vi "YAFFooter_TemplateMethod.vi"(8 "ErrorIn":errorcluster, 10 "CmdData":variant, 11 "YAFFooter:YAFFooter in":refnum<class>) -> (0 "ErrorOut":errorcluster, 2 "ReplyData":variant, 3 "YAFFooter:YAFFooter out":refnum<class>, 4 "Exit":bool)   [LabVIEW 2021, in "YAFFooter.lvlib" / "YAFFooter.lvclass"]
uses:
  YAFFooter.lvclass
  YAFFooter.lvclass/YAFFooter.ctl
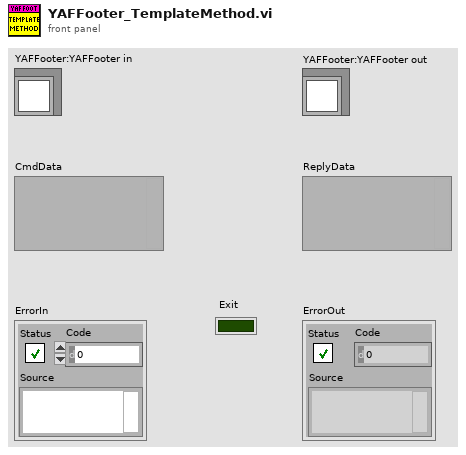
[diagram p1: front panel]
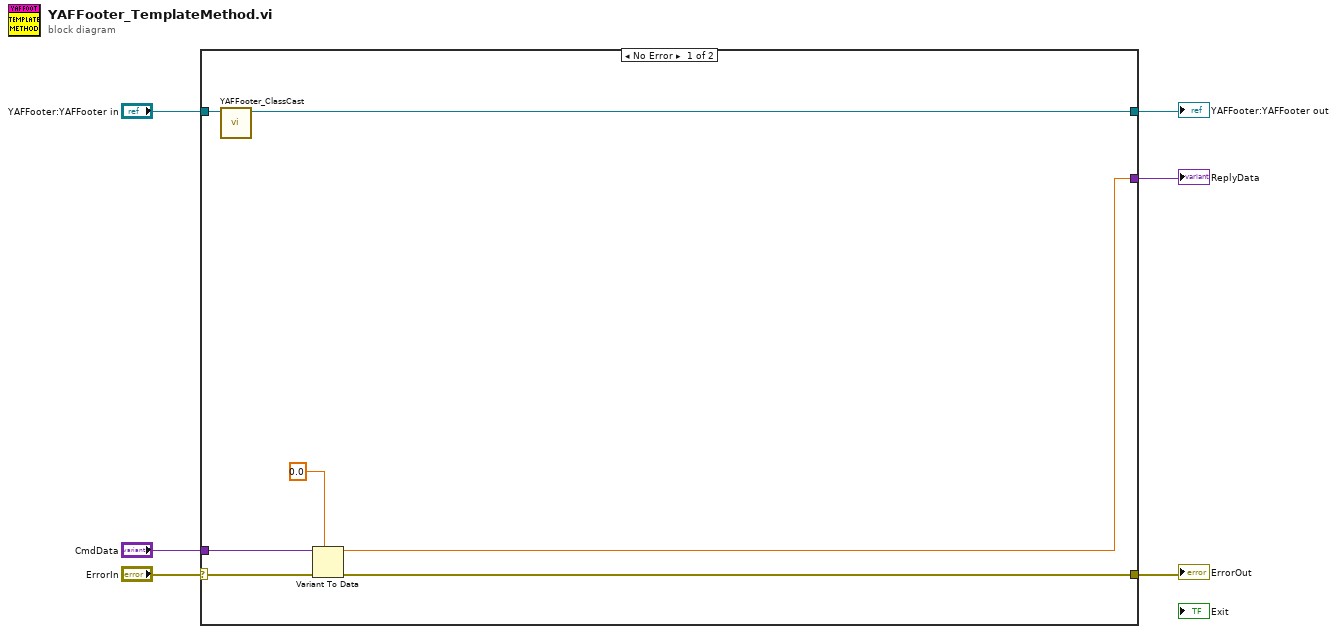
[diagram p0: block diagram]
diagram:
  n1 = case shown="No Error" "ErrorIn" {
    selector: "ErrorIn" -> [w13 w16]
    tunnel: [w12 w16] -> w5
    tunnel: [w7 w15] -> w3
    tunnel: "CmdData" -> [w10 w15]
    tunnel: "YAFFooter:YAFFooter in" -> [w11 w14]
    tunnel: [w9 w14] -> w1
    frame No Error {
      n2 = call "YAFFooter_ClassCast.vi"("YAFFooter:YAFFooter in"=w11) -> ("YAFFooter:YAFFooter out"=w9:refnum<class "YAFFooter.lvclass">)  [unwired: 10 in]
      n3 = Variant To Data(error in=w13, type=0.0 ("DummyIn"), Variant=w10) -> (data=w7:dbl, error out=w12:errorcluster)
    }
    frame Error {
    }
  }
  "ErrorOut" <- w5
  "YAFFooter:YAFFooter out" <- w1
  "ReplyData" <- w3
